vi "Read Section Names and Keys.vi"(8 "error in (no error)":errorcluster, 11 "Configuration in":refnum<class "Configuration.lvclass">) -> (0 "error out":errorcluster, 2 "Sections":T1(array[cluster]), 3 "Configuration out":refnum<class "Configuration.lvclass">)   [LabVIEW 2014, in "Configuration.lvlib" / "Configuration.lvclass"]
doc: "Read configuration data from class private data."
uses:
  Configuration.lvclass
  Configuration.lvclass/Configuration.ctl
  Section/Section.lvclass
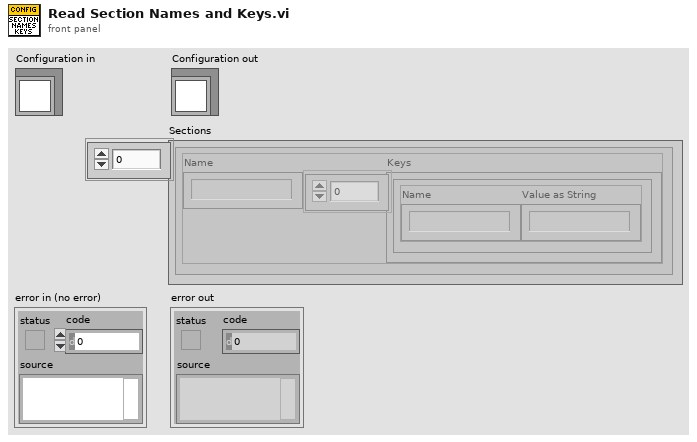
[diagram p1: front panel]
types:
  T1 = cluster{"Name":string, "Keys":cluster{"Name":string, "Value as String":string}[]}[]
  T2 = cluster{"Name":string, "Keys":cluster{"Name":string, "Value":string}[]}
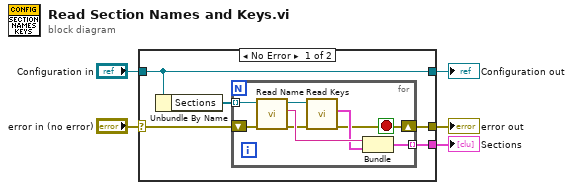
[diagram p0: block diagram]
diagram:
  n1 = case shown="No Error" "error in (no error)" {
    selector: "error in (no error)" -> [w7 w20]
    tunnel: [w6 w20] -> w4
    tunnel: [w10 w19] -> w2
    tunnel: "Configuration in" -> [w10 w19]
    tunnel: [w8 _] -> w1
    frame No Error {
      n2 = Unbundle By Name(w10) -> ("Sections"=w9:refnum<class "Section.lvclass">[])
      n3 = for {
        tunnel: w9 -> [w18] mode=indexing
        tunnel: [w16] -> w8 mode=indexing
        shift-right: [w11] -> w6
        shift-left: w7 -> [w12]
        stop <- w11 stop-if-true
        n4 = call "Read Name.vi"("error in (no error)"=w12, "Section in"=w18) -> ("error out"=w14:errorcluster, "Name"=w17:string, "Section out"=w15:refnum<class "Section.lvclass">)  [unwired: 7 in]
        n5 = call-dynamic "Read Keys.vi"("error in (no error)"=w14, "Section in"=w15) -> ("error out"=w11:errorcluster, "Keys"=w13:cluster{"Name":string, "Value":string}[])  [unwired: 7 in, 1 out]
        n6 = Bundle("Name"=w17, "Keys"=w13) -> (w16:T2)  [unwired: 1 in]
      }
    }
    frame Error {
    }
  }
  "error out" <- w4
  "Configuration out" <- w2
  "Sections" <- w1
